vi "SW Interface - SET - Triggered Events & Data.vi"(8 "error in (no error)":errorcluster, 9 "Data":string, 10 "Events":T1, 11 "Child_2_Class in":refnum<class "SW_Interface_Class.lvclass">) -> (0 "error out":errorcluster, 3 "Child_2_Class out":refnum<class "SW_Interface_Class.lvclass">)   [LabVIEW 2023, in "SW_Interface_Actor.lvlib" / "SW_Interface_Class.lvclass"]
uses:
  SW_Interface_Class.lvclass
  Usr Ev/SW Interface - Ctrl - Enum - Events (Temp).ctl
  SW_Interface_Class.lvclass/SW_Interface_Class.ctl
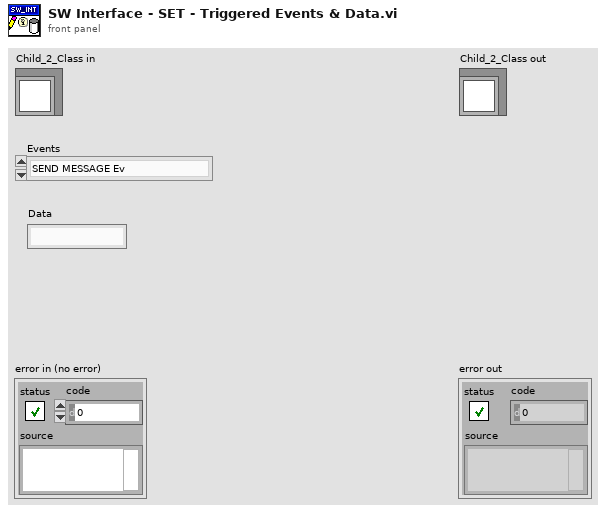
[diagram p1: front panel]
types:
  T1 = typedef "SW_Interface_Actor.lvlib/SW_Interface_Class.lvclass/SW Interface - Ctrl - Enum - Events (Temp).ctl" = enum16{"SEND MESSAGE Ev", "STOP_ACTOR Ev", "INIT_ACTOR Ev", "START Ev", "STOP Ev", "GET Ev", "SET Ev", "ERROR_HANDLER Ev", "RESET Ev", "T2 Ev", "T3 Ev", "T4 Ev"}
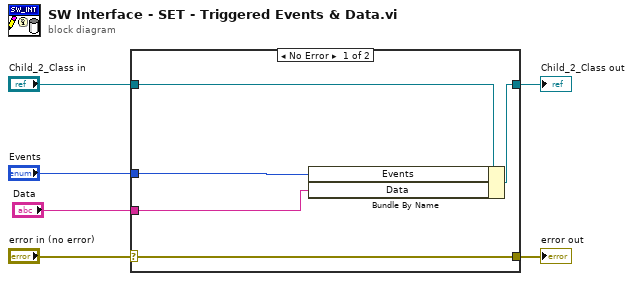
[diagram p0: block diagram]
diagram:
  n1 = case shown="No Error" "error in (no error)" {
    selector: "error in (no error)" -> [w11 w12]
    tunnel: [w11 w12] -> w5
    tunnel: [w9 w13] -> w3
    tunnel: "Child_2_Class in" -> [w10 w13]
    tunnel: "Events" -> [w8 _]
    tunnel: "Data" -> [w7 _]
    frame No Error {
      n2 = Bundle By Name(cluster=w10, "Events"=w8, "Data"=w7) -> (w9:refnum<class "SW_Interface_Class.lvclass">)
    }
    frame Error {
    }
  }
  "error out" <- w5
  "Child_2_Class out" <- w3
